vi "Read Get Laser Status.lvclass.vi"(8 "error in (no error)":errorcluster, 11 "In":refnum<class "Recipe View.lvclass">) -> (0 "error out":errorcluster, 2 "Get Laser Status.lvclass":refnum<class "Get Laser Status.lvclass">, 3 "Out":refnum<class "Recipe View.lvclass">)   [LabVIEW 2022 SP3, in "Recipe View.lvclass"]
uses:
  Recipe View.lvclass
  Recipe View.lvclass/Recipe View.ctl
  Laser/Get Laser Status/Get Laser Status.lvclass
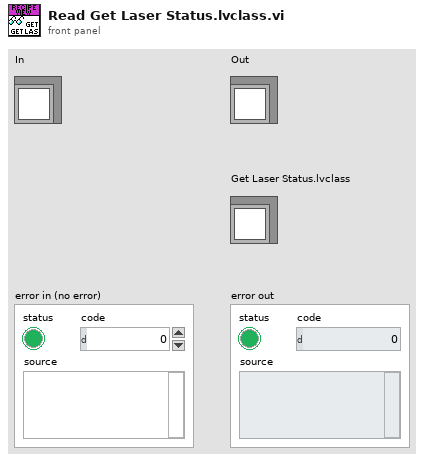
[diagram p1: front panel]
types:
  T1 = typedef "Recipe View.lvclass/Data.ctl" = cluster{"Recipe API.lvclass":refnum<class "Recipe API.lvclass">, "XY stage VIEW":refnum<class "base view.lvclass">, "Laser VIEW":refnum<class "base view.lvclass">, "Camera VIEW":refnum<class "base view.lvclass">, "DAQ VIEW":refnum<class "base view.lvclass">, "Stop":refnum<user-event>, "Camera Async Coms.lvclass":refnum<class "Camera Async Coms.lvclass">, "Get Daq Status.lvclass":refnum<class "Get Daq Status.lvclass">, "Get Laser Status.lvclass":refnum<class "Get Laser Status.lvclass">, "2-Axis Stage Status.lvclass":refnum<class "2-Axis Stage Status.lvclass">}
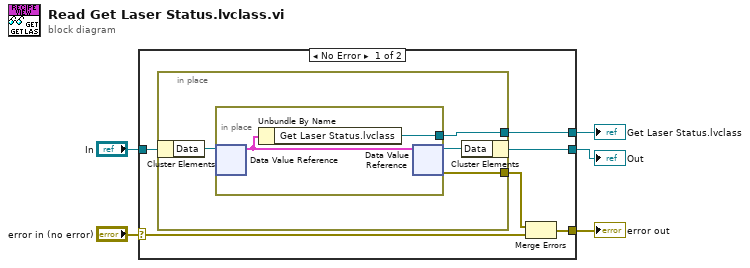
[diagram p0: block diagram]
diagram:
  n1 = case shown="No Error" "error in (no error)" {
    selector: "error in (no error)" -> [w6 w19]
    tunnel: [w7 w19] -> w4
    tunnel: [w11 w18] -> w3
    tunnel: "In" -> [w10 w18]
    tunnel: [w9 _] -> w1
    frame No Error {
      n2 = in-place {
        in-place-border: [w13] -> w9
        in-place-border: [w12] -> w8
        n3 = in-place-cluster #1(w10) -> ("Data"=w14:refnum<data-value>)
        n4 = in-place {
          in-place-border: [w16] -> w13
          n5 = in-place-dvr #2(w14) -> (w17:T1)  [unwired: 1 out]
          n6 = Unbundle By Name(w17) -> ("Get Laser Status.lvclass"=w16:refnum<class "Get Laser Status.lvclass">)
          n7 = in-place-dvr #2(w17) -> (w15:refnum<data-value>, w12:errorcluster)
        }
        n8 = in-place-cluster #1("Data"=w15) -> (w11:refnum<class "Recipe View.lvclass">)
      }
      n9 = Merge Errors(w8, w6) -> (w7:errorcluster)
    }
    frame Error {
    }
  }
  "Out" <- w3
  "error out" <- w4
  "Get Laser Status.lvclass" <- w1
